vi "Processamento.vi"(7 "error in":errorcluster) -> ()   [LabVIEW 2017]
uses:
  <vilib>/vision/Contour.llb/IMAQ Contour Curve Extraction.ctl
  <vilib>/vision/NI_Vision_Development_Module.lvlib
panel:
  out "XY Graph":cluster{"X":dbl, "Y":dbl}[](graph)
  out "Number of Objects":i32
  out "Image Out":T1(plugin-control)
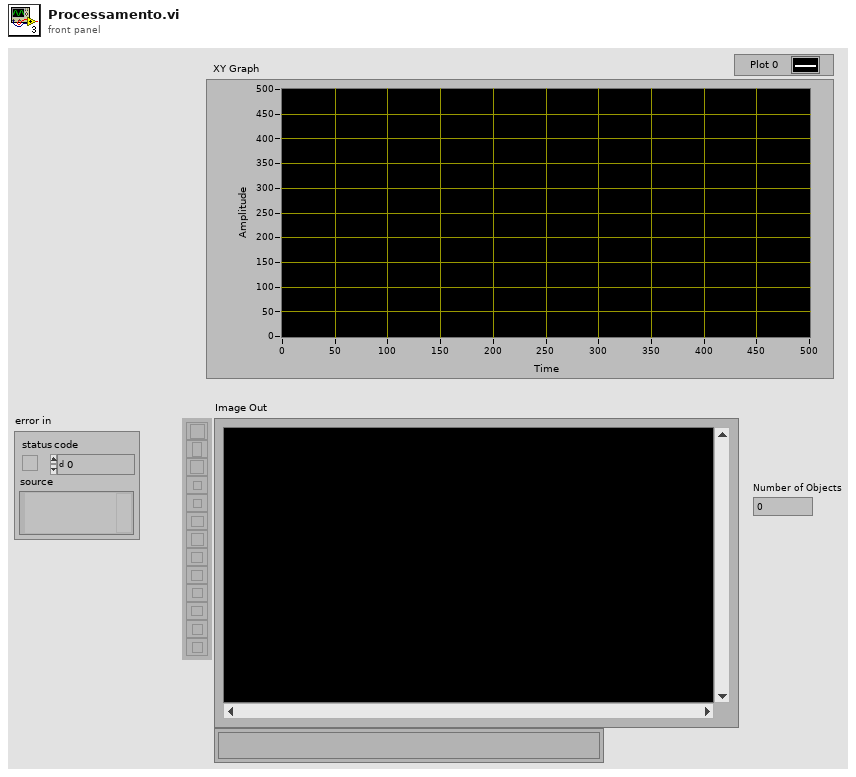
[diagram p1: front panel]
types:
  T1 = typedef "IMAQ Image.ctl" = refnum<image>
  T2 = cluster{"Objects":u16, "Threshold":i32, "Reject Border":bool, "Fill Holes":bool, "Min Object Size":bool, "Min Size":i32, "Max Object Size":bool, "Max Size":i32, "Show Search Area":bool, "Show Center":bool, "Show Bounding Box":bool}
  T3 = enum32{"AutoM", "Close", "Dilate", "Erode", "Gradient", "Gradient out", "Gradient in", "Hit miss", "Open", "PClose", "POpen", "Thick", "Thin"}
  T4 = cluster{"Global Rectangle":i32[], "Contours":cluster{"ID":enum32{"External", "Internal"}, "Type":u32, "Coordinates":i32[]}[]}
  T5 = typedef "Image Type" = u32
  T6 = cluster{"Object Center":cluster{"X":sgl, "Y":sgl}, "Bounding Box":cluster{"X Left":i32, "Y Top":i32, "X Right":i32, "Y Bottom":i32}, "Area":sgl, "Orientation":sgl, "Aspect Ratio":sgl, "Nb Holes":i32}[]
  T7 = enum16{"Rect Left To Right", "Rect Right To Left", "Rect Top To Bottom", "Rect Bottom To Top", "Annulus Inner To Outer", "Annulus Outer To Inner", "Annulus Start Angle To End Angle", "Annulus End Angle To Start Angle"}
  T8 = enum16{"Closest To Search Start", "Maximum Length", "Strongest Mean Gradient Change"}
  T9 = typedef "IMAQ Contour Curve Extraction.ctl" = cluster{"Extraction Mode":u32, "Edge Threshold":i32, "Edge Filter Size":u32, "Min Length":i32, "Search Step Size":i32, "Max Endpoint Gap":i32, "Subpixel":bool}
  T10 = cluster{"Object Center":cluster{"X":sgl, "Y":sgl}, "Bounding Box":cluster{"X Left":i32, "Y Top":i32, "X Right":i32, "Y Bottom":i32}, "Area":sgl, "Orientation":sgl, "Aspect Ratio":sgl, "Nb Holes":i32}
  T11 = cluster{"X Left":i32, "Y Top":i32, "X Right":i32, "Y Bottom":i32, dbl}
  T12 = typedef "ROI Descriptor" = cluster{"Global Rectangle":i32[], "Contours":cluster{"ID":enum32{"External", "Internal"}, "Type":u32, "Coordinates":i32[]}[]}
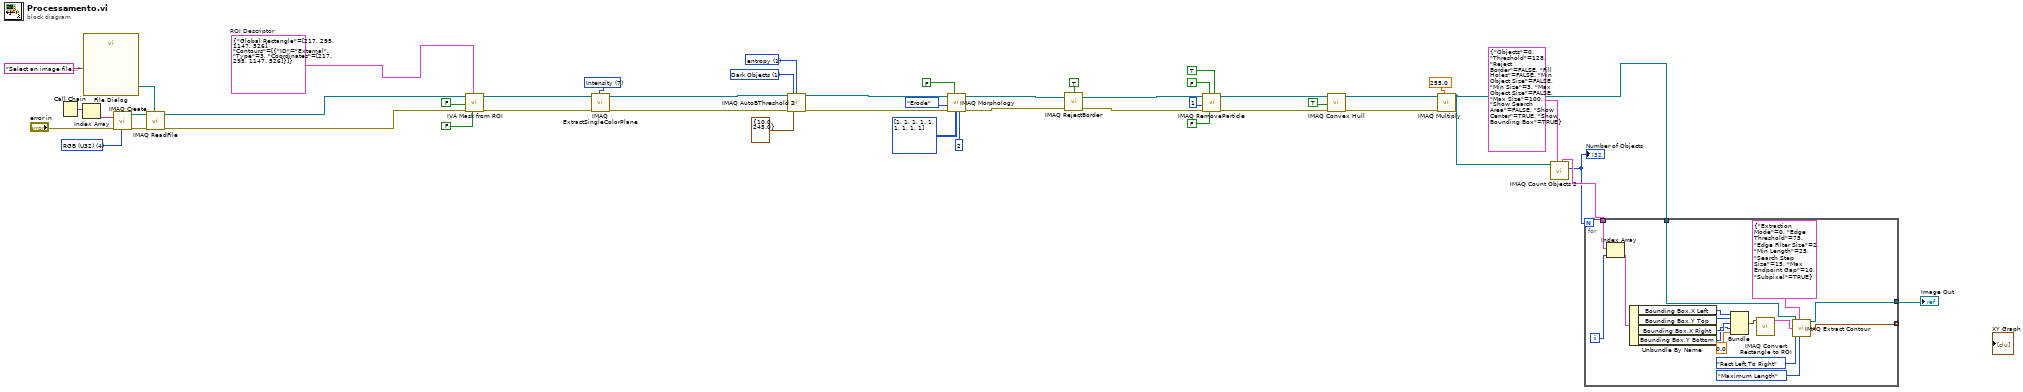
[diagram p0: block diagram]
diagram:
  w27 = 1 items=["clustering", "entropy", "metric", "moments", "inter-class variance"] ("Method")
  w28 = u32 1 items=["Bright Objects", "Dark Objects"] ("Look For")
  w33 = 7 items=["Red", "Green", "Blue", "Hue", "Saturation", "Luminance", "Value", "Intensity"] ("Color Plane")
  w38 = T4 {"Global Rectangle"=[217, 295, 1147, 526], "Contours"=[{"ID"=enum."External", "Type"=3, "Coordinates"=[217, 295, 1147, 526]}]}  # ROI Descriptor
  w39 = T5 4 items=["Grayscale (U8)", "Grayscale (I16)", "Grayscale (SGL)", "Complex (CSG)", "RGB (U32)", "HSL (U32)", "RGB (U64)", "Grayscale (U16)"] ("Image Type")
  n1 = Call Chain() -> (call chain=w43:string[])
  n2 = Index Array(array=w43) -> (element=w42:string)  [unwired: 1 in]
  n3 = call "File Dialog"("prompt"="Select an image file...") -> ("selected path"=w40:path)  [unwired: 6 in, 8 out]
  n4 = call "IMAQ Create"("Image Name"=w42, "Image Type"=w39, "error in (no error)"="error in") -> ("New Image"=w46:T1, "error out"=w45:errorcluster)  [unwired: 1 in, 1 out]
  n5 = call "IMAQ ReadFile"("File Path"=w40, "error in (no error)"=w45, "Image"=w46) -> ("error out"=w47:errorcluster, "Image Out"=w36:T1)  [unwired: 2 in, 5 out]
  n6 = call <vilib>:"IVA Mask from ROI.vi"("Shrink"=FALSE, "ROI Descriptor"=w38, "error in (no error)"=w47, "Out / In"=FALSE, "Image Src"=w36) -> ("error out"=w34:errorcluster, "Image Out"=w32:T1)  [unwired: 5 out]
  n7 = call "IMAQ ExtractSingleColorPlane"("Color Plane"=w33, "error in (no error)"=w34, "Image Src"=w32) -> ("error out"=w31:errorcluster, "Image Dst Out"=w30:T1)  [unwired: 1 in, 6 out]
  n8 = call "IMAQ AutoBThreshold 2"("Image Src"=w30, "Look For (Bright Objects)"=w28, "Method (clustering)"=w27, "error in (no error)"=w31, "Threshold Limits"=cluster{"Lower value":sgl, "Upper value":sgl} {"Lower value"=10.0, "Upper value"=245.0}) -> ("Image Dst Out"=w21:T1, "error out"=w29:errorcluster)  [unwired: 3 in, 6 out]
  n9 = call "IMAQ Morphology"("Number of iterations (1)"=2, "Structuring Element"=i32[][] [[1, 1, 1], [1, 1, 1], [1, 1, 1]], "Square/Hexa (Square)"=FALSE, "error in (no error)"=w29, "Operation"=T3."Erode", "Image Src"=w21) -> ("error out"=w20:errorcluster, "Image Dst Out"=w18:T1)  [unwired: 1 in, 3 out]
  n10 = call "IMAQ RejectBorder"("error in (no error)"=w20, "Image Src"=w18, "Connectivity 4/8 (8)"=TRUE) -> ("error out"=w17:errorcluster, "Image Dst Out"=w12:T1)  [unwired: 1 in, 2 out]
  n11 = call "IMAQ RemoveParticle"("Connectivity 4/8 (8)"=TRUE, "Low Pass/High Pass (Low)"=FALSE, "Square/Hexa (Square)"=FALSE, "error in (no error)"=w17, "Number of Erosion"=1, "Image Src"=w12) -> ("error out"=w11:errorcluster, "Image Dst Out"=w10:T1)  [unwired: 1 in, 3 out]
  n12 = call "IMAQ Convex Hull"("error in (no error)"=w11, "Connectivity 4/8 (8)"=TRUE, "Image Src"=w10) -> ("error out"=w8:errorcluster, "Image Dst Out"=w6:T1)  [unwired: 1 in, 6 out]
  n13 = call "IMAQ Multiply"("Image Src A"=w6, "Constant"=sgl 255.0, "error in (no error)"=w8) -> ("Image Dst Out"=w3:T1)  [unwired: 2 in, 3 out]
  n14 = call "IMAQ Count Objects 2"("Settings"=T2 {"Objects"=0, "Threshold"=128, "Reject Border"=FALSE, "Fill Holes"=FALSE, "Min Object Size"=FALSE, "Min Size"=3, "Max Object Size"=FALSE, "Max Size"=100, "Show Search Area"=FALSE, "Show Center"=TRUE, "Show Bounding Box"=TRUE}, "Image"=w3) -> ("Number of Objects"=w4:i32, "Objects"=w5:T6)  [unwired: 5 in, 3 out]
  "Number of Objects" <- w4
  n15 = for {
    N: w4 -> [_]
    tunnel: w5 -> [w63]
    tunnel: w3 -> [w51]
    tunnel: [w50] -> w2
    tunnel: [w48] -> _ mode=indexing
    i -> [w49]
    n16 = Index Array(array=w63, index=w49) -> (element=w62:T10)
    n17 = Unbundle By Name(w62) -> ("Bounding Box.X Left"=w57:i32, "Bounding Box.Y Top"=w56:i32, "Bounding Box.X Right"=w55:i32, "Bounding Box.Y Bottom"=w54:i32)
    n18 = Bundle("X Left"=w57, "Y Top"=w56, "X Right"=w55, "Y Bottom"=w54, 0.0) -> (w52:T11)  [unwired: 1 in]
    n19 = call "IMAQ Convert Rectangle to ROI"("Rectangle"=w52) -> ("ROI Descriptor"=w59:T12)  [unwired: 8 in, 1 out]
    n20 = call "IMAQ Extract Contour"("Source Image"=w51, "Curve Extraction"=T9 {"Extraction Mode"=0, "Edge Threshold"=75, "Edge Filter Size"=2, "Min Length"=25, "Search Step Size"=15, "Max Endpoint Gap"=10, "Subpixel"=TRUE}, "ROI Descriptor"=w59, "Search Direction"=T7."Rect Left To Right", "Contour Selection"=T8."Maximum Length") -> ("Source Image Out"=w50:T1, "Contour Points"=w48:cluster{"X":dbl, "Y":dbl}[])  [unwired: 3 in, 6 out]
  }
  "Image Out" <- w2
